vi "Main2.vi"() -> ()   [LabVIEW 2014]
uses:
  Framework/Base.lvclass
panel:
  in  "vi path":path
  out "class name":string
  out "class path":path
  out "error out":errorcluster
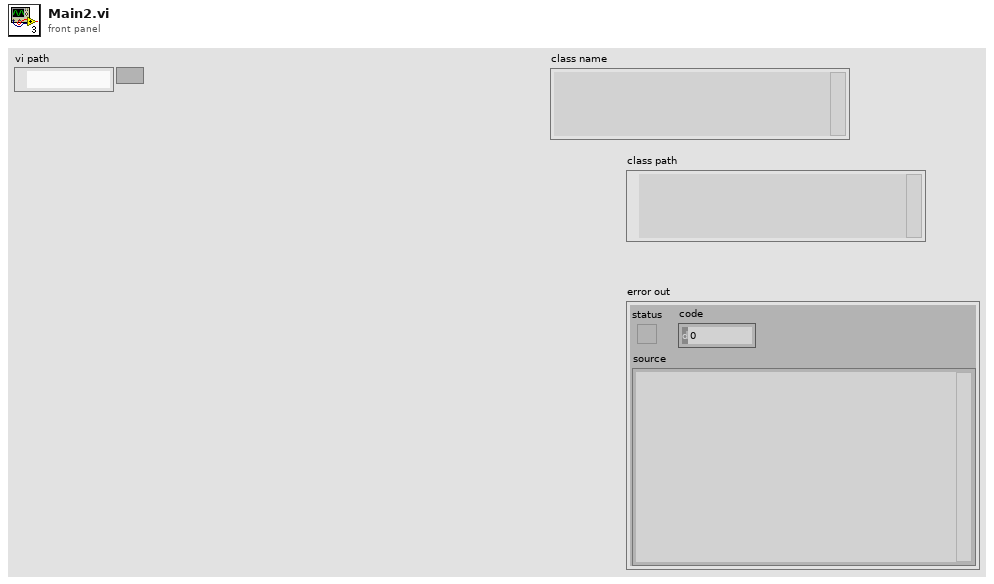
[diagram p1: front panel]
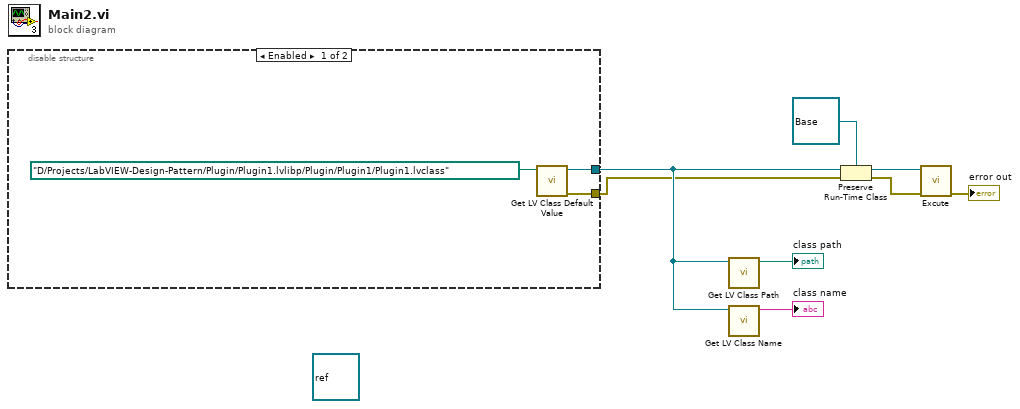
[diagram p0: block diagram]
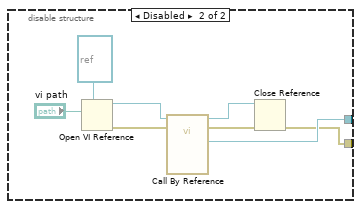
[diagram p2: hidden frame]
diagram:
  (unwired) refnum<class> refnum ("LabVIEW Object")
  n1 = disable-structure shown="Enabled" {
    disable-tunnel: [w11 w13] -> w2
    disable-tunnel: [w10 w15] -> w5
    frame Enabled {
      n2 = call <vilib>:"Get LV Class Default Value.vi"("class path"=path "D:/Projects/LabVIEW-Design-Pattern/Plugin/Plugin1.lvlibp/Plugin/Plugin1/Plugin1.lvclass" ("class path 2")) -> ("error out"=w11:errorcluster, "object"=w10:refnum<class>)  [unwired: 9 in]
    }
    frame Disabled {
      n3 = Open VI Reference(type specifier VI Refnum (for type only)=refnum<vi> refnum, vi path="vi path") -> (vi reference=w18:refnum<vi>, error out=w19:errorcluster)  [unwired: 4 in]
      n4 = call-by-ref "?"(reference=w18, error in=w19) -> (reference out=w12:refnum<vi>, error out=w14:errorcluster, "Plugin"=w15:refnum<class "Base.lvclass">)  [unwired: 11 in]
      n5 = Close Reference(reference=w12, error in (no error)=w14) -> (error out=w13:errorcluster)
    }
  }
  n6 = call <vilib>:"Get LV Class Path.vi"("object"=w5) -> ("class path"=→"class path":path)  [unwired: 9 in, 1 out]
  n7 = call <vilib>:"Get LV Class Name.vi"("object"=w5) -> ("class name"=→"class name":string)  [unwired: 9 in, 1 out]
  n8 = Preserve Run-Time Class(object in=w5, error in=w2, 2:refnum<class "Base.lvclass"> refnum ("Framework.lvlib:Base.lvclass")) -> (object out=w3:refnum<class "Base.lvclass">, error out=w1:errorcluster)
  n9 = call-dynamic "Excute.vi"("error in (no error)"=w1, "Base in"=w3) -> ("error out"=→"error out":errorcluster)  [unwired: 8 in, 1 out]
